vi "Handle.vi"(10 "Msg":refnum<class "Msg.lvclass">, 11 "Actor in":refnum<class "Actor.lvclass">) -> (0 "Error out":errorcluster, 3 "Actor out":refnum<class "Actor.lvclass">)   [LabVIEW 2020, in "jettl.lvlib" / "Actor.lvlib" / "Actor.lvclass"]
uses:
  Actor.lvclass
  Msg/Msg.lvclass
  Attributes/Attributes/Attributes.lvclass
  Actor.lvlib
  Error/Error.lvlib
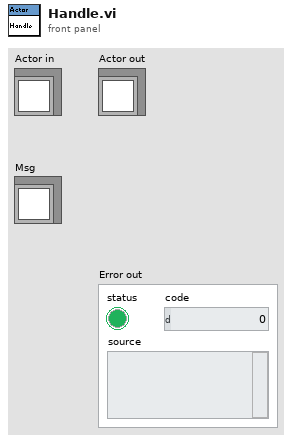
[diagram p1: front panel]
types:
  T1 = typedef "jettl.lvlib/Actor.lvlib/Msg Set.ctl" = set{refnum<class "Msg.lvclass">}
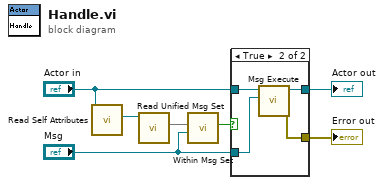
[diagram p0: block diagram]
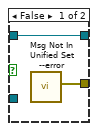
[diagram p2: hidden frame]
diagram:
  n1 = call-dynamic "Read Self Attributes.vi"("Actor in"="Actor in") -> ("Self Attributes"=w7:refnum<class "Attributes.lvclass">)  [unwired: 10 in]
  n2 = call-dynamic "Read Unified Msg Set.vi"("Attributes in"=w7) -> ("Unified Msg Set"=w6:T1)  [unwired: 10 in]
  n3 = call "Within Msg Set.vi"("Msg"="Msg", "Msg Set"=w6) -> ("Within Msg Set"=w4:bool)  [unwired: 9 in]
  n4 = case shown="True" w4 {
    tunnel: "Actor in" -> [w9 w13]
    tunnel: [w9 w12] -> w2
    tunnel: "Msg" -> [_ w11]
    tunnel: [w8 w10] -> w1
    frame False {
      n5 = call "Msg Not In Unified Set --error.vi"() -> ("Error"=w8:errorcluster)  [unwired: 11 in]
    }
    frame True {
      n6 = call-dynamic "Msg Execute.vi"("Msg"=w11, "Actor in"=w13) -> ("Error out"=w10:errorcluster, "Actor out"=w12:refnum<class "Actor.lvclass">)  [unwired: 8 in]
    }
  }
  "Actor out" <- w2
  "Error out" <- w1
